vi "Delete Block Diagram Objects.vi"(8 "error in (no error)":errorcluster, 11 "Owner in":refnum<vi>) -> (0 "error out":errorcluster, 3 "Owner out":refnum<vi>)   [LabVIEW 2018, in "Scripting.lvlib"]
uses:
  Scripting.lvlib
  <vilib>/Utility/traverseref.llb/TRef TravTarget.ctl
  <vilib>/Utility/traverseref.llb/VI Scripting - Traverse.lvlib
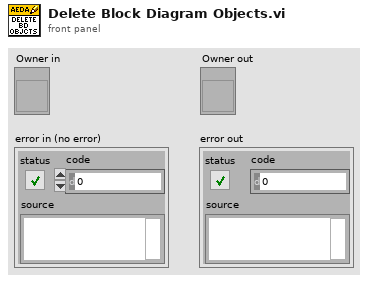
[diagram p1: front panel]
types:
  T1 = typedef "TRef TravTarget.ctl" = enum16{"FP", "BD", "Other"}
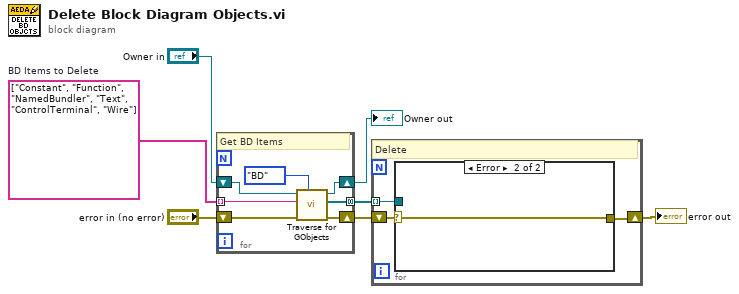
[diagram p0: block diagram]
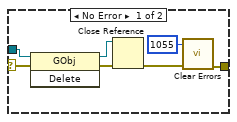
[diagram p2: hidden frame]
diagram:
  w6 = string[] ["Constant", "Function", "NamedBundler", "Text", "ControlTerminal", "Wire"]  # BD Items to Delete
  n1 = for {
    tunnel: [w12] -> w3 mode=concatenating
    shift-right: [w13] -> w2
    shift-left: "error in (no error)" -> [w14]
    shift-right: [w10] -> w7
    shift-left: "Owner in" -> [w11]
    tunnel: w6 -> [w9] mode=indexing
    # "Get BD Items"
    n2 = call <vilib>:"Traverse for GObjects.vi"("Traverse Target"=TRef_TravTarget."BD", "error in (no error)"=w14, "Class Name"=w9, "VI Refnum"=w11) -> ("error out"=w13:errorcluster, "References"=w12:refnum<vi>[], "dup VI Refnum"=w10:refnum<vi>)  [unwired: 4 in, 1 out]
  }
  "Owner out" <- w7
  n3 = for {
    tunnel: w3 -> [w17] mode=indexing
    shift-right: [w15] -> w5
    shift-left: w2 -> [w16]
    # "Delete"
    n4 = case shown="Error" w16 {
      selector: w16 -> [w23 w25]
      tunnel: w17 -> [w24 _]
      tunnel: [w18 w25] -> w15
      frame No Error {
        n5 = invoke class="GObj" method="Delete"(reference=w24, error in=w23) -> (reference out=w21:refnum<vi>, error out=w22:errorcluster)  [unwired: 1 in, 1 out]
        n6 = Close Reference(reference=w21, error in (no error)=w22) -> (error out=w20:errorcluster)
        n7 = call <vilib>:"Clear Errors.vi"("error in (no error)"=w20, "specific error code to clear (0: all)"=1055) -> ("error out"=w18:errorcluster)  [unwired: 4 in, 1 out]
      }
      frame Error {
      }
    }
  }
  "error out" <- w5
